vi "goToPoint.vi"() -> (0 "y result":dbl=0.011895720106726845, 3 "x result":dbl=0.10938578018522986)   [LabVIEW 2020]
uses:
  Robot Global Data.vi
  <vilib>/addons/control/pid/pid.llb/PID (DBL).vi
  <vilib>/addons/control/pid/NI_PID_pid.lvlib
panel:
  in  "y gains":T1={"proportional gain (Kc)"=-0.4, "integral time (Ti, min)"=0.0, "derivative time (Td, min)"=0.0} {"derivative time (Td, min)" format="%.25f"; "integral time (Ti, min)" format="%.25f"; "proportional gain (Kc)" format="%.25f"}
  in  "x gains":T1={"proportional gain (Kc)"=-0.5, "integral time (Ti, min)"=0.0, "derivative time (Td, min)"=0.0} {"derivative time (Td, min)" format="%.25f"; "integral time (Ti, min)" format="%.25f"; "proportional gain (Kc)" format="%.25f"}
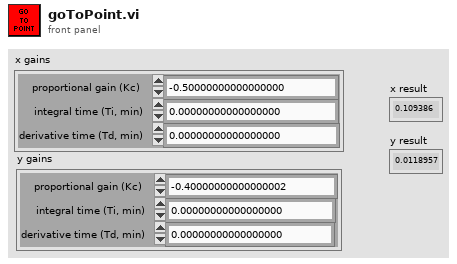
[diagram p1: front panel]
types:
  T1 = cluster{"proportional gain (Kc)":dbl, "integral time (Ti, min)":dbl, "derivative time (Td, min)":dbl}
  T2 = cluster{"POSE.TRANSLATION.X":dbl, "POSE.TRANSLATION.Y":dbl}
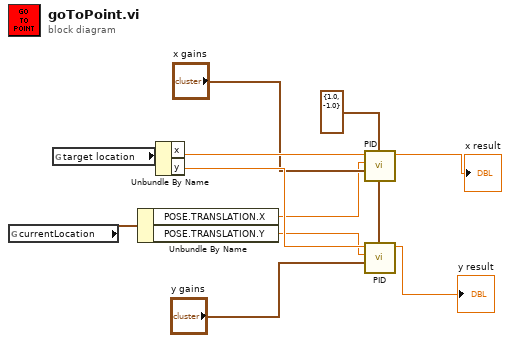
[diagram p0: block diagram]
diagram:
  w10 = cluster{"output high":dbl, "output low":dbl} {"output high"=1.0, "output low"=-1.0} ("output range")
  n1 = global read "Robot Global Data.vi" "currentLocation"() -> (w5:T2)
  n2 = global read "Robot Global Data.vi" "target location"() -> (w11:cluster{"x":dbl, "y":dbl})
  n3 = Unbundle By Name(w5) -> ("POSE.TRANSLATION.X"=w3:dbl, "POSE.TRANSLATION.Y"=w4:dbl)
  n4 = Unbundle By Name(w11) -> ("x"=w9:dbl, "y"=w8:dbl)
  n5 = call-poly <vilib>:"PID.vi"("output range"=w10, "PID gains"="x gains", "process variable"=w3, "setpoint"=w9) -> ("output"=→"x result":dbl)  [unwired: 6 in, 1 out]
  n6 = call-poly <vilib>:"PID.vi"("output range"=w10, "PID gains"="y gains", "process variable"=w4, "setpoint"=w8) -> ("output"=→"y result":dbl)  [unwired: 6 in, 1 out]
